vi "NI DAQ Channels.vi"(4 "Control":bool, 6 "Channel":string, 7 "AO Data":dbl format="%0.2f", 8 "error in (no error)":errorcluster, 10 "Path":path, 11 "Command":string) -> (0 "error out":errorcluster, 3 "Pressure":dbl)   [LabVIEW 2015]
uses:
  Controls/Channel Info.ctl
  <vilib>/DAQmx/read.llb/DAQmx Read (Analog DBL 1Chan 1Samp).vi
  <vilib>/DAQmx/write.llb/DAQmx Write (Digital Bool 1Line 1Point).vi
  <vilib>/DAQmx/write.llb/DAQmx Write (Analog DBL 1Chan 1Samp).vi
  <vilib>/DAQmx/miscellaneous.llb/DAQmx Fill In Error Info.vi
  <vilib>/Utility/file.llb/Read Delimited Spreadsheet (string).vi
  <vilib>/DAQmx/create/channels.llb/DAQmx Create Channel (DO-Digital Output).vi
  <vilib>/DAQmx/create/channels.llb/DAQmx Create Channel (AO-Current-Basic).vi
  <vilib>/DAQmx/create/channels.llb/DAQmx Create Channel (AI-Current-Basic).vi
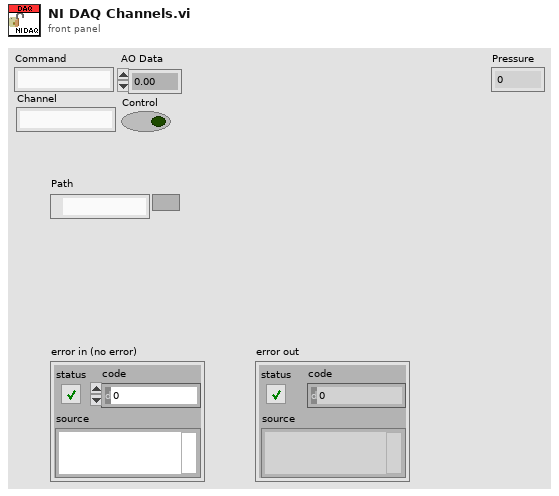
[diagram p1: front panel]
types:
  T1 = typedef "Channel Info.ctl" = cluster{"Channel":string, "Type":string, "Task":refnum<k21>}
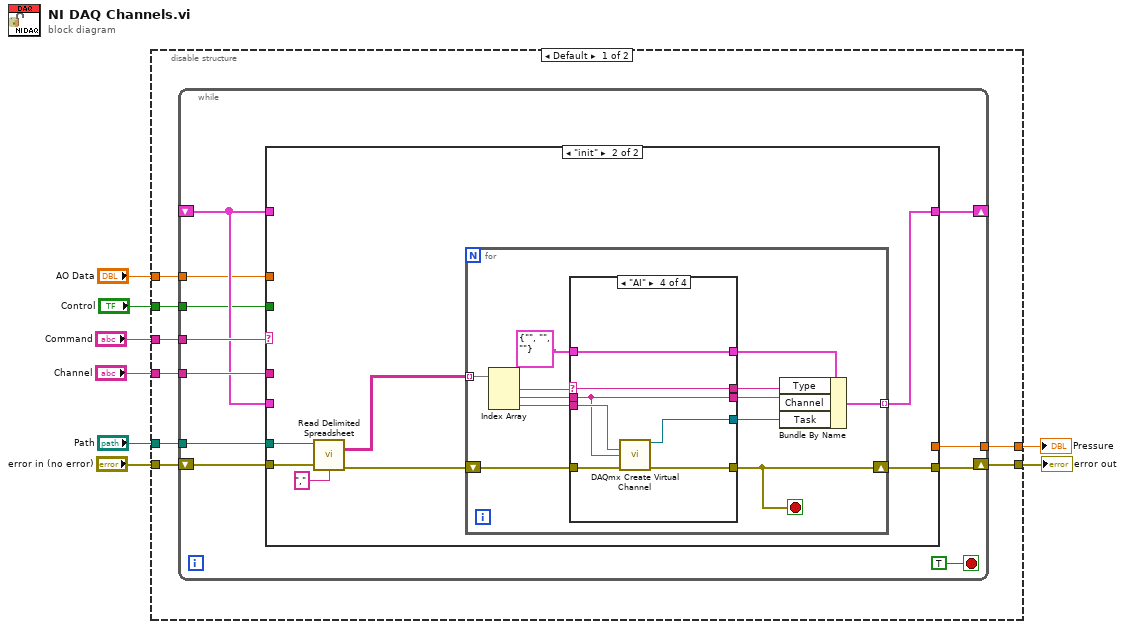
[diagram p0: block diagram]
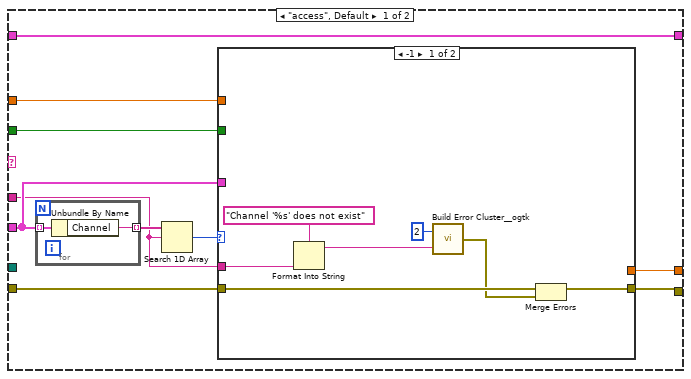
[diagram p2: hidden frame]
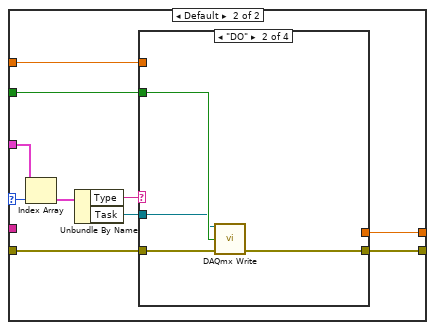
[diagram p3: hidden frame]
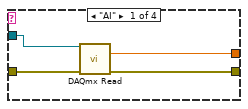
[diagram p4: hidden frame]
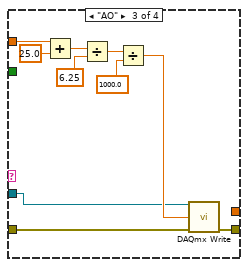
[diagram p5: hidden frame]
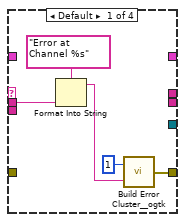
[diagram p7: hidden frame]
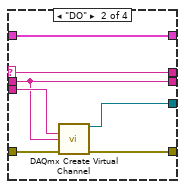
[diagram p8: hidden frame]
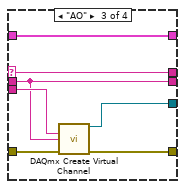
[diagram p9: hidden frame]
diagram:
  n1 = disable-structure shown="Default" {
    disable-tunnel: "Command" -> [w16 _]
    disable-tunnel: "error in (no error)" -> [w15 w121]
    disable-tunnel: [w14 w121] -> w6
    disable-tunnel: "Path" -> [w13 _]
    disable-tunnel: "Channel" -> [w12 _]
    disable-tunnel: "AO Data" -> [w11 _]
    disable-tunnel: [w10 _] -> w2
    disable-tunnel: "Control" -> [w9 _]
    frame condition #0 (active) {
      n2 = while {
        tunnel: w16 -> [w26]
        shift-right: [w23] -> w14
        shift-left: w15 -> [w25]
        tunnel: w13 -> [w24]
        shift-right: [w22] -> _
        shift-left: _ -> [w20]
        tunnel: w12 -> [w21]
        tunnel: w11 -> [w19]
        tunnel: [w18] -> w10
        tunnel: w9 -> [w17]
        stop <- TRUE stop-if-true
        n3 = case shown="\"init\"" w26 {
          tunnel: w25 -> [w36 w81]
          tunnel: w24 -> [_ w82]
          tunnel: [w34 w77] -> w23
          tunnel: [w37 w76] -> w22
          tunnel: w20 -> [w29 _]
          tunnel: w21 -> [w28 _]
          tunnel: w20 -> [w37 _]
          tunnel: w19 -> [w35 _]
          tunnel: [w33 _] -> w18
          tunnel: w17 -> [w32 _]
          frame "access", Default {
            n4 = for {
              tunnel: w29 -> [w75] mode=indexing
              tunnel: [w74] -> w31 mode=indexing
              n5 = Unbundle By Name(w75) -> ("Channel"=w74:string)
            }
            n6 = Search 1D Array(1D array=w31, element=w28) -> (index of element=w30:i32)  [unwired: 1 in]
            n7 = case shown="-1" w30 {
              selector: w30 -> [_ w49]
              tunnel: w36 -> [w40 w54]
              tunnel: w35 -> [_ w53]
              tunnel: [w38 w52] -> w34
              tunnel: [_ w51] -> w33
              tunnel: w32 -> [_ w50]
              tunnel: w29 -> [_ w48]
              tunnel: w28 -> [w43 _]
              frame -1 {
                n8 = Format Into String(format string="Channel '%s' does not exist", w43) -> (resulting string=w41:string)  [unwired: 2 in, 1 out]
                n9 = call <userlib>:"Build Error Cluster__ogtk.vi"("String to Prepend to source (\"\")"=w41, "code"=2) -> ("error out"=w39:errorcluster)
                n10 = Merge Errors(w40, w39) -> (w38:errorcluster)
              }
              frame Default {
                n11 = Index Array(array=w48, index=w49) -> (element=w47:T1)
                n12 = Unbundle By Name(w47) -> ("Type"=w46:string, "Task"=w45:refnum<k21>)
                n13 = case shown="\"DO\"" w46 {
                  tunnel: w54 -> [w58 w62 w72 w73]
                  tunnel: w53 -> [_ _ w70 _]
                  tunnel: [w57 w61 w71 w73] -> w52
                  tunnel: [w56 _ _ _] -> w51
                  tunnel: w50 -> [_ w60 _ _]
                  tunnel: w45 -> [w55 w59 w63 _]
                  frame "AI" {
                    n14 = call-poly <vilib>:"DAQmx Read.vi"("task/channels in"=w55, "error in"=w58) -> ("data"=w56:dbl, "error out"=w57:errorcluster)  [unwired: 11 in, 1 out]
                  }
                  frame "DO" {
                    n15 = call-poly <vilib>:"DAQmx Write.vi"("task/channels in"=w59, "data"=w60, "error in"=w62) -> ("error out"=w61:errorcluster)  [unwired: 10 in, 2 out]
                  }
                  frame "AO" {
                    n16 = Add(x=w70, y=25.0) -> (x+y=w68:dbl)
                    n17 = Divide(x=w68, y=6.25) -> (x/y=w66:dbl)
                    n18 = Divide(x=w66, y=1000.0) -> (x/y=w64:dbl)
                    n19 = call-poly <vilib>:"DAQmx Write.vi"("task/channels in"=w63, "data"=w64, "error in"=w72) -> ("error out"=w71:errorcluster)  [unwired: 10 in, 2 out]
                  }
                  frame Default {
                  }
                }
              }
            }
          }
          frame "init" {
            n20 = call-poly <vilib>:"Read Delimited Spreadsheet.vi"("file path (dialog if empty)"=w82, "error in (no error)"=w81, "delimiter (\\t)"="," ("delimiter (\\t)")) -> ("all rows"=w78:string[][], "error out"=w79:errorcluster)  [unwired: 7 in, 4 out]
            n21 = for {
              shift-right: [w88] -> w77
              shift-left: w79 -> [w90]
              tunnel: w78 -> [w94] mode=indexing
              tunnel: [w83] -> w76 mode=indexing
              stop <- w88 stop-if-true
              n22 = Index Array(array=w94) -> (element #1=w93:string, element #2=w91:string, element #3=w89:string)  [unwired: 3 in]
              n23 = case shown="\"AI\"" w93 {
                selector: w93 -> [_ w102 w109 w116]
                tunnel: T1 {"Channel"="", "Type"="", "Task"=""} ("Channel Info") -> [_ w103 w110 w117]
                tunnel: w91 -> [w97 w101 w108 w115]
                tunnel: w90 -> [_ w106 w113 w120]
                tunnel: w89 -> [_ w105 w112 w119]
                tunnel: [w99 w104 w111 w118] -> w88
                tunnel: [_ w103 w110 w117] -> w87
                tunnel: [_ w102 w109 w116] -> w86
                tunnel: [_ w101 w108 w115] -> w85
                tunnel: [_ w100 w107 w114] -> w84
                frame Default {
                  n24 = Format Into String(format string="Error at Channel %s", w97) -> (resulting string=w95:string)  [unwired: 2 in, 1 out]
                  n25 = call <userlib>:"Build Error Cluster__ogtk.vi"("String to Prepend to source (\"\")"=w95, "code"=1) -> ("error out"=w99:errorcluster)
                }
                frame "DO" {
                  n26 = call-poly <vilib>:"DAQmx Create Virtual Channel.vi"("lines"=w105, "name to assign"=w101, "error in"=w106) -> ("task out"=w100:refnum<k21>, "error out"=w104:errorcluster)  [unwired: 11 in]
                }
                frame "AO" {
                  n27 = call-poly <vilib>:"DAQmx Create Virtual Channel.vi"("physical channels"=w112, "name to assign"=w108, "error in"=w113) -> ("task out"=w107:refnum<k21>, "error out"=w111:errorcluster)  [unwired: 11 in]
                }
                frame "AI" {
                  n28 = call-poly <vilib>:"DAQmx Create Virtual Channel.vi"("physical channels"=w119, "name to assign"=w115, "error in"=w120) -> ("task out"=w114:refnum<k21>, "error out"=w118:errorcluster)  [unwired: 11 in]
                }
              }
              n29 = Bundle By Name(cluster=w87, "Type"=w86, "Channel"=w85, "Task"=w84) -> (w83:T1)
            }
          }
        }
      }
    }
    frame condition #1 {
    }
  }
  "error out" <- w6
  "Pressure" <- w2
